vi "9219_GetStrValMappings.vi"(1 "_Include \"invalid\" Range item (F)":bool, 2 "_Include \"invalid\" Range2 item (F)":bool, 3 "_Include \"invalid\" RTD (F)":bool, 5 "_Mode":u8) -> (6 "_Mode (str)":string, 8 "_Range Strings And Values []":cluster{"String":string, "Value":u16}[](array[cluster]), 10 "_Range2 Strings And Values []":cluster{"String":string, "Value":u16}[](array[cluster]), 15 "_RTD Strings And Values []":cluster{"String":string, "Value":u16}[](array[cluster]))   [LabVIEW 2011, in "Modules.lvlib" / "9219.lvclass"]
uses:
  9219.lvclass
panel:
  out "RTD Type Typedef":u8(ring) items=["TCR3851"=1, "TCR3750"=2, "TCR3916"=3, "TCR3920"=4, "TCR3911"=5, "TCR3928"=6, "Custom"=0]
  out "Thermocouple Typedef":u8(ring) items=["J", "K", "T", "E", "R", "S", "N", "B"]
  out "Degree Range Typedef":u8(ring) items=["Raw units", "Degrees Kelvin", "Degrees Celsius", "Degrees Fahrenheit", "Degrees Rankine"]
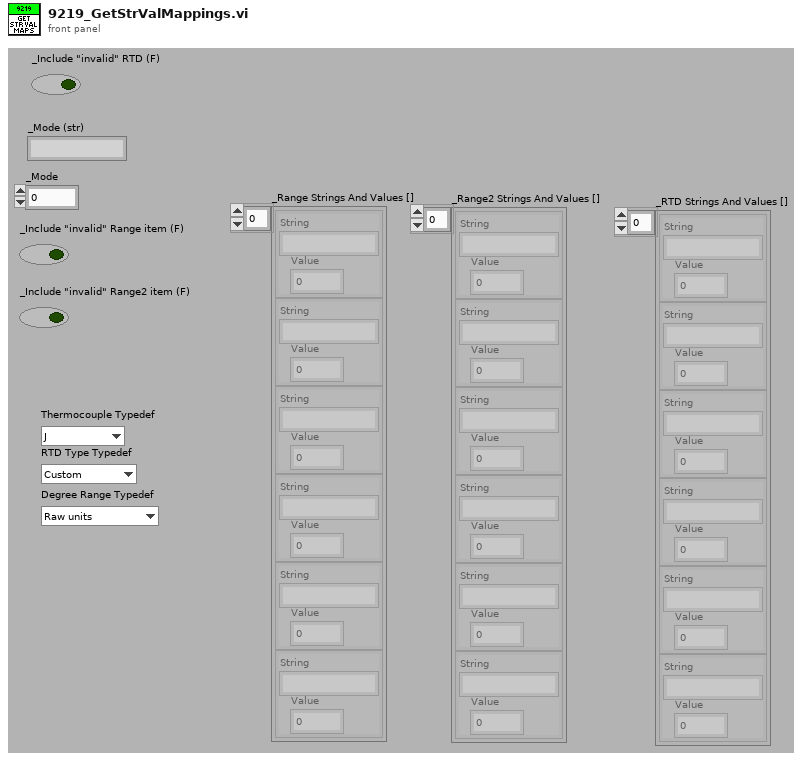
[diagram p1: front panel]
types:
  T1 = typedef "LVStringsAndValuesArrayTypeDef.ctl" = cluster{"String":string, "Value":u8}[]
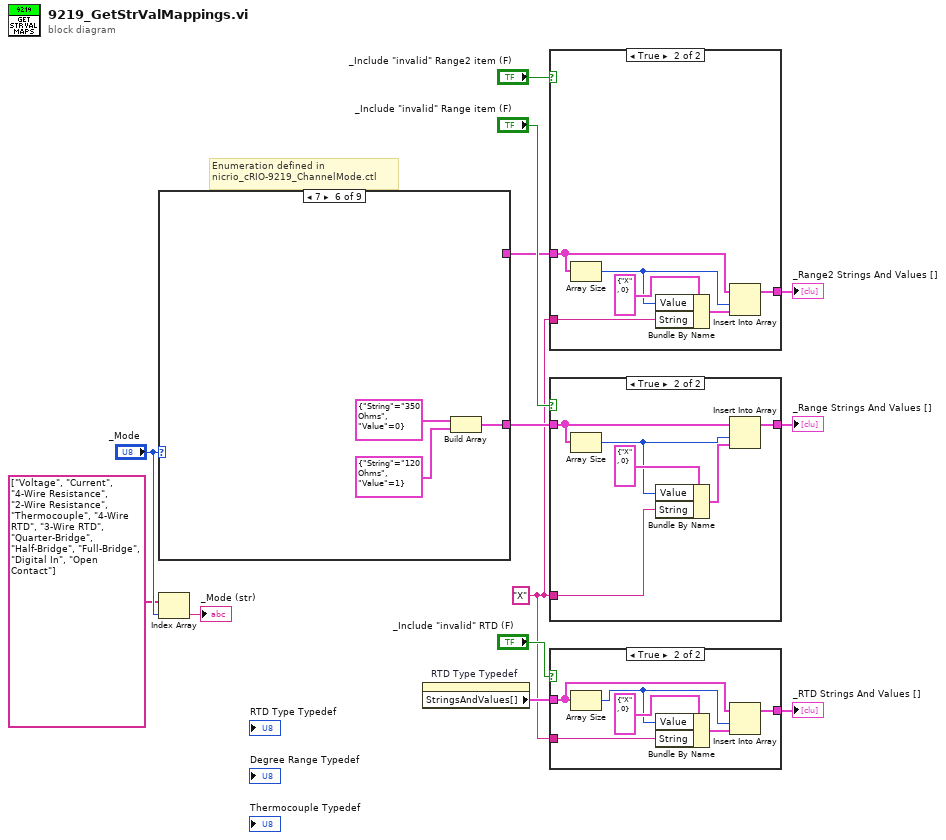
[diagram p0: block diagram]
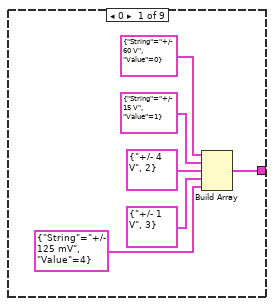
[diagram p5: hidden frame]
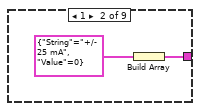
[diagram p6: hidden frame]
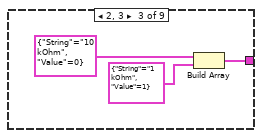
[diagram p7: hidden frame]
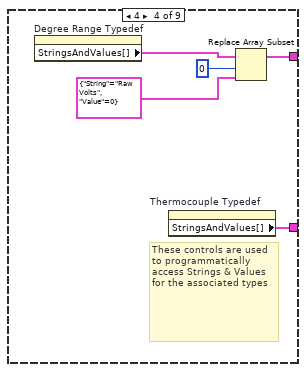
[diagram p8: hidden frame]
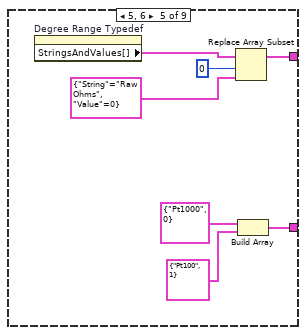
[diagram p9: hidden frame]
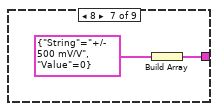
[diagram p10: hidden frame]
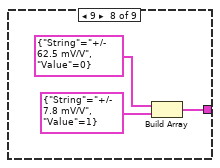
[diagram p11: hidden frame]
diagram:
  w1 = "X" ("String")
  # "Enumeration defined in \nnicrio_cRIO-9219_ChannelMode.ctl"
  n1 = case shown="7" "_Mode" {
    tunnel: [w19 w21 w24 w29 w36 w39 w41 w44 _] -> w10
    tunnel: [_ _ _ w28 w35 _ _ _ _] -> w6
    frame 0 {
      n2 = Build Array(cluster{"String":string, "Value":u16} {"String"="+/- 60 V", "Value"=0}, cluster{"String":string, "Value":u16} {"String"="+/- 15 V", "Value"=1}, cluster{"String":string, "Value":u16} {"String"="+/- 4 V", "Value"=2}, cluster{"String":string, "Value":u16} {"String"="+/- 1 V", "Value"=3}, cluster{"String":string, "Value":u16} {"String"="+/- 125 mV", "Value"=4}) -> (w19:cluster{"String":string, "Value":u16}[])
    }
    frame 1 {
      n3 = Build Array(cluster{"String":string, "Value":u16} {"String"="+/- 25 mA", "Value"=0}) -> (w21:cluster{"String":string, "Value":u16}[])
    }
    frame 2, 3 {
      n4 = Build Array(cluster{"String":string, "Value":u16} {"String"="10 kOhm", "Value"=0}, cluster{"String":string, "Value":u16} {"String"="1 kOhm", "Value"=1}) -> (w24:cluster{"String":string, "Value":u16}[])
    }
    frame 4 {
      # "These controls are used to programmatically access Strings & Values for the associated types"
      n5 = property on="Degree Range Typedef" class="Ring (strict)"() -> ("StringsAndValues[]"=w27:T1)  [unwired: 2 in, 2 out]
      n6 = property on="Thermocouple Typedef" class="Ring (strict)"() -> ("StringsAndValues[]"=w29:T1)  [unwired: 2 in, 2 out]
      n7 = Replace Array Subset(array=w27, new element=cluster{"String":string, "Value":u16} {"String"="Raw Volts", "Value"=0}, index=0) -> (w28:T1)
    }
    frame 5, 6 {
      n8 = property on="Degree Range Typedef" class="Ring (strict)"() -> ("StringsAndValues[]"=w34:T1)  [unwired: 2 in, 2 out]
      n9 = Replace Array Subset(array=w34, new element=cluster{"String":string, "Value":u16} {"String"="Raw Ohms", "Value"=0}, index=0) -> (w35:T1)
      n10 = Build Array(cluster{"String":string, "Value":u16} {"String"="Pt1000", "Value"=0}, cluster{"String":string, "Value":u16} {"String"="Pt100", "Value"=1}) -> (w36:cluster{"String":string, "Value":u16}[])
    }
    frame 7 {
      n11 = Build Array(cluster{"String":string, "Value":u16} {"String"="350 Ohms", "Value"=0}, cluster{"String":string, "Value":u16} {"String"="120 Ohms", "Value"=1}) -> (w39:cluster{"String":string, "Value":u16}[])
    }
    frame 8 {
      n12 = Build Array(cluster{"String":string, "Value":u16} {"String"="+/- 500 mV/V", "Value"=0}) -> (w41:cluster{"String":string, "Value":u16}[])
    }
    frame 9 {
      n13 = Build Array(cluster{"String":string, "Value":u16} {"String"="+/- 62.5 mV/V", "Value"=0}, cluster{"String":string, "Value":u16} {"String"="+/- 7.8 mV/V", "Value"=1}) -> (w44:cluster{"String":string, "Value":u16}[])
    }
    frame Default {
      # "No Str-Val mappings for other modes"
    }
  }
  n14 = Index Array(array=string[] ["Voltage", "Current", "4-Wire Resistance", "2-Wire Resistance", "Thermocouple", "4-Wire RTD", "3-Wire RTD", "Quarter-Bridge", "Half-Bridge", "Full-Bridge", "Digital In", "Open Contact"], index="_Mode") -> (element=→"_Mode (str)":string)
  n15 = property on="RTD Type Typedef" class="Ring (strict)"() -> ("StringsAndValues[]"=w3:T1)  [unwired: 2 in, 2 out]
  n16 = case shown="True" "_Include \"invalid\" Range2 item (F)" {
    tunnel: w6 -> [w45 w51]
    tunnel: [w45 w50] -> w7
    tunnel: w1 -> [_ w46]
    frame False {
    }
    frame True {
      n17 = Array Size(array=w51) -> (size(s)=w47:i32)
      n18 = Bundle By Name(cluster=cluster{"String":string, "Value":u16} {"String"="X", "Value"=0}, "Value"=w47, "String"=w46) -> (w48:cluster{"String":string, "Value":u16})
      n19 = Insert Into Array(array=w51, index=w47, new element=w48) -> (w50:T1)
    }
  }
  "_Range2 Strings And Values []" <- w7
  n20 = case shown="True" "_Include \"invalid\" Range item (F)" {
    tunnel: w10 -> [w52 w58]
    tunnel: [w52 w57] -> w9
    tunnel: w1 -> [_ w53]
    frame False {
    }
    frame True {
      n21 = Array Size(array=w58) -> (size(s)=w54:i32)
      n22 = Bundle By Name(cluster=cluster{"String":string, "Value":u16} {"String"="X", "Value"=0}, "Value"=w54, "String"=w53) -> (w55:cluster{"String":string, "Value":u16})
      n23 = Insert Into Array(array=w58, index=w54, new element=w55) -> (w57:cluster{"String":string, "Value":u16}[])
    }
  }
  "_Range Strings And Values []" <- w9
  n24 = case shown="True" "_Include \"invalid\" RTD (F)" {
    tunnel: w3 -> [w59 w65]
    tunnel: [w59 w64] -> w5
    tunnel: w1 -> [_ w60]
    frame False {
    }
    frame True {
      n25 = Array Size(array=w65) -> (size(s)=w61:i32)
      n26 = Bundle By Name(cluster=cluster{"String":string, "Value":u16} {"String"="X", "Value"=0}, "Value"=w61, "String"=w60) -> (w62:cluster{"String":string, "Value":u16})
      n27 = Insert Into Array(array=w65, index=w61, new element=w62) -> (w64:T1)
    }
  }
  "_RTD Strings And Values []" <- w5
